vi "PCTuidToDB.vi"(8 "error in":errorcluster caption="错误输入（无错误）", 9 "TuidName":string="4G T-BOX.txt", 10 "CertName":string="证书列表.txt", 11 "PathStr":string) -> (0 "error out":errorcluster caption="错误输出", 3 "OK？":bool)   [LabVIEW 2013]
panel:
  out "连接的字符串":string
  out "数组":string[](array[string])
  out "TUID":string[](array[string])
  out "TUID":string
  out "证书":string[](array[string])
  out "Certificate":string
  out "添加的路径":path
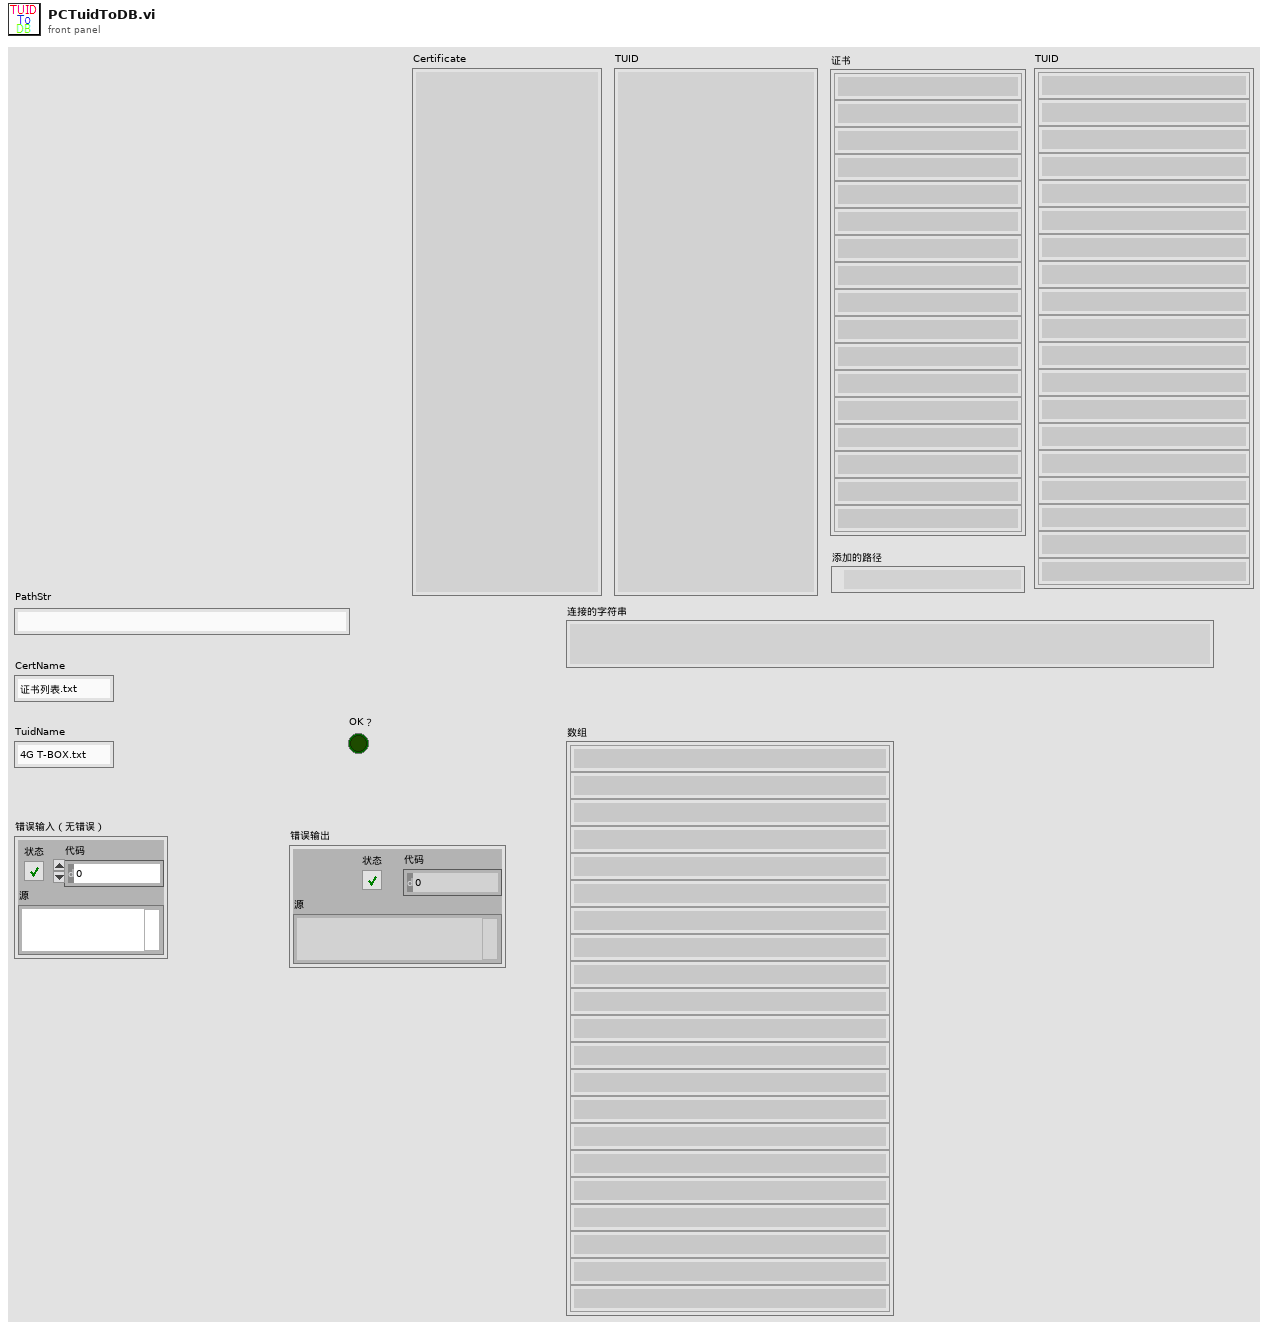
[diagram p1: front panel]
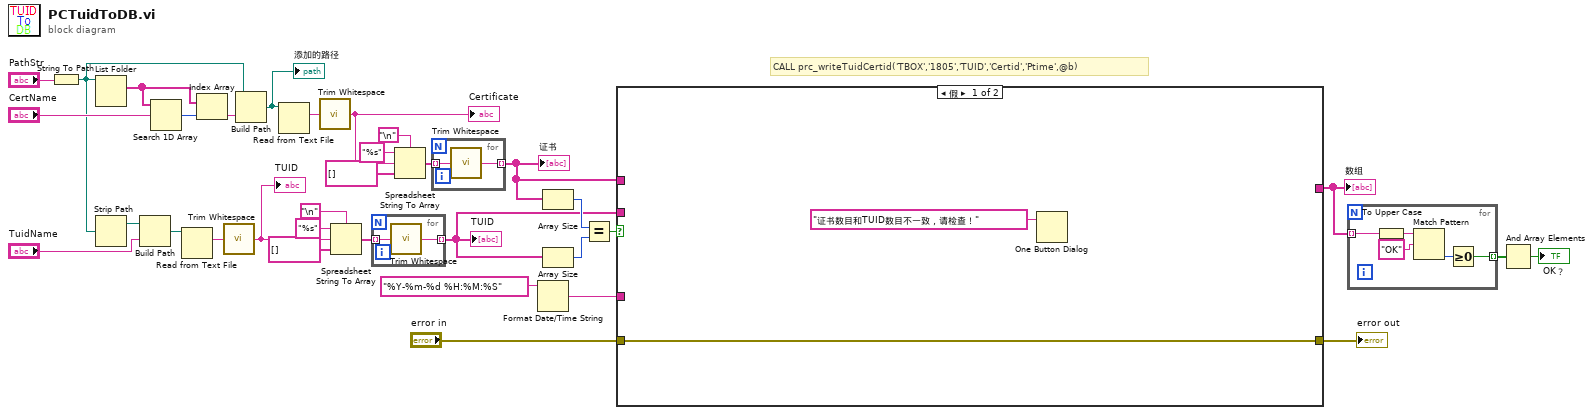
[diagram p0: block diagram]
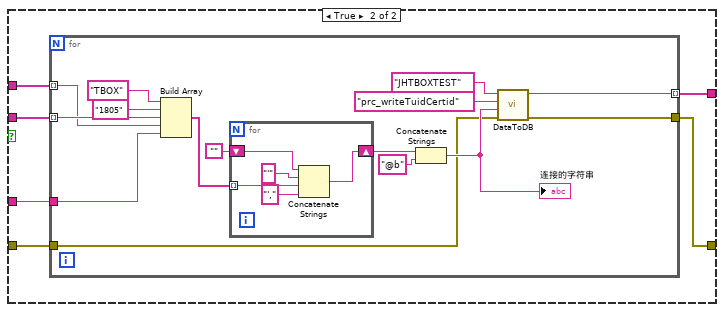
[diagram p2: hidden frame]
diagram:
  # "CALL prc_writeTuidCertid('TBOX','1805','TUID','Certid','Ptime',@b)"
  n1 = String To Path(string="PathStr") -> (path=w10:path)
  n2 = List Folder(path=w10) -> (filenames=w33:string[])  [unwired: 3 in, 3 out]
  n3 = Strip Path(path=w10) -> (stripped path=w25:path)  [unwired: 1 out]
  n4 = Build Path(base path=w25, name or relative path="TuidName") -> (appended path=w23:path)
  n5 = Search 1D Array(1D array=w33, element="CertName") -> (index of element=w32:i32)  [unwired: 1 in]
  n6 = Read from Text File(file (use dialog)=w23) -> (text=w19:string)  [unwired: 3 in, 3 out]
  n7 = Index Array(array=w33, index=w32) -> (element=w31:string)
  n8 = call <vilib>:"Trim Whitespace.vi"("string"=w19) -> ("trimmed string"=w13:string)  [unwired: 1 in]
  "TUID" <- w13
  n9 = Build Path(base path=w10, name or relative path=w31) -> (appended path=w30:path)
  "添加的路径" <- w30
  n10 = Read from Text File(file (use dialog)=w30) -> (text=w28:string)  [unwired: 3 in, 3 out]
  n11 = call <vilib>:"Trim Whitespace.vi"("string"=w28) -> ("trimmed string"=w12:string)  [unwired: 1 in]
  "Certificate" <- w12
  n12 = Spreadsheet String To Array(delimiter (Tab)="\n", format string="%s" ("格式字符串"), spreadsheet string=w13, array type (2D Dbl)=string[] []) -> (array=w2:string[])
  n13 = for {
    tunnel: w2 -> [w36] mode=indexing
    tunnel: [w35] -> w1 mode=indexing
    n14 = call <vilib>:"Trim Whitespace.vi"("string"=w36) -> ("trimmed string"=w35:string)  [unwired: 1 in]
  }
  "TUID" <- w1
  n15 = Spreadsheet String To Array(delimiter (Tab)="\n", format string="%s" ("格式字符串"), spreadsheet string=w12, array type (2D Dbl)=string[] []) -> (array=w4:string[])
  n16 = for {
    tunnel: w4 -> [w38] mode=indexing
    tunnel: [w37] -> w3 mode=indexing
    n17 = call <vilib>:"Trim Whitespace.vi"("string"=w38) -> ("trimmed string"=w37:string)  [unwired: 1 in]
  }
  "证书" <- w3
  n18 = Format Date/Time String(time format string (%c)="%Y-%m-%d %H:%M:%S" ("Procedure name")) -> (date/time string=w14:string)  [unwired: 2 in]
  n19 = Array Size(array=w3) -> (size(s)=w18:i32)
  n20 = Array Size(array=w1) -> (size(s)=w17:i32)
  n21 = Equal?(x=w18, y=w17) -> (x = y?=w16:bool)
  n22 = case shown="假" w16 {
    tunnel: w1 -> [_ w43]
    tunnel: w3 -> [_ w44]
    tunnel: [_ w46] -> w7
    tunnel: w14 -> [_ w45]
    tunnel: "error in" -> [w39 w42]
    tunnel: [w39 w41] -> w8
    frame False {
      n23 = One Button Dialog(message="证书数目和TUID数目不一致，请检查！" ("消息")) -> ()  [unwired: 1 in, 1 out]
    }
    frame True {
      n24 = for {
        tunnel: [w59] -> w46 mode=indexing
        tunnel: w45 -> [w49]
        tunnel: w44 -> [w50] mode=indexing
        tunnel: w43 -> [w51] mode=indexing
        tunnel: [w47] -> w41
        tunnel: w42 -> [w48]
        n25 = Build Array("TBOX" ("Procedure name"), "1805" ("Procedure name"), w51, w50, w49) -> (w55:string[])
        n26 = for {
          shift-right: [w62] -> w54
          shift-left: "" -> [w66]
          tunnel: w55 -> [w65] mode=indexing
          n27 = Concatenate Strings(w66, "'", w65, "',") -> (w62:string)
        }
        n28 = Concatenate Strings(w54, "@b" ("字符串")) -> (w52:string)
        "连接的字符串" <- w52
        n29 = call "DataToDB.vi"("error in"=w48, "all string"=w52, "Procedure name"="prc_writeTuidCertid", "DSN name"="JHTBOXTEST") -> ("error out"=w47:errorcluster, "ReportStrA"=w59:string)  [unwired: 4 in, 2 out]
      }
    }
  }
  "数组" <- w7
  "error out" <- w8
  n30 = for {
    tunnel: w7 -> [w71] mode=indexing
    tunnel: [w67] -> w6 mode=indexing
    n31 = To Upper Case(1:w71) -> (0:w70:string)
    n32 = Match Pattern(string=w70, regular expression="OK") -> (offset past match=w68:i32)  [unwired: 1 in, 3 out]
    n33 = Greater Or Equal To 0?(x=w68) -> (x >= 0?=w67:bool)
  }
  n34 = And Array Elements(Boolean array=w6) -> (logical AND=→"OK？":bool)
